vi "seriesName.set.vi"(8 "error in (no error)":errorcluster, 10 "seriesName":string, 11 "timestampMetadata in":refnum<class "timestampMetadata.lvclass">) -> (0 "error out":errorcluster, 3 "timestampMetadata out":refnum<class "timestampMetadata.lvclass">)   [LabVIEW 2020, in "timestampMetadata.lvclass"]
uses:
  timestampMetadata.lvclass
  timestampMetadata.lvclass/timestampMetadata.ctl
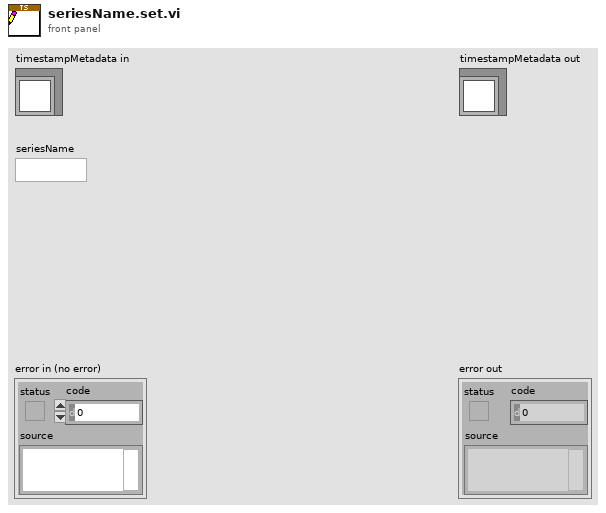
[diagram p1: front panel]
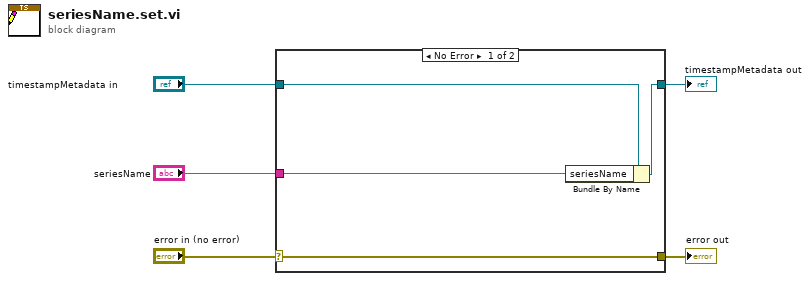
[diagram p0: block diagram]
diagram:
  n1 = case shown="No Error" "error in (no error)" {
    selector: "error in (no error)" -> [w9 w10]
    tunnel: [w9 w10] -> w4
    tunnel: [w7 w11] -> w2
    tunnel: "timestampMetadata in" -> [w8 w11]
    tunnel: "seriesName" -> [w6 _]
    frame No Error {
      n2 = Bundle By Name(cluster=w8, "seriesName"=w6) -> (w7:refnum<class "timestampMetadata.lvclass">)
    }
    frame Error {
    }
  }
  "error out" <- w4
  "timestampMetadata out" <- w2
